vi "Dialog.vi"(8 "error in (no error)":errorcluster, 10 "latest tag":string, 11 "SelfUpdate in":refnum<class "SelfUpdate.lvclass">) -> (0 "error out":errorcluster, 2 "T button?":bool, 3 "SelfUpdate out":refnum<class "SelfUpdate.lvclass">)   [LabVIEW 2013, in "SelfUpdate.lvclass"]
uses:
  SelfUpdate.lvclass
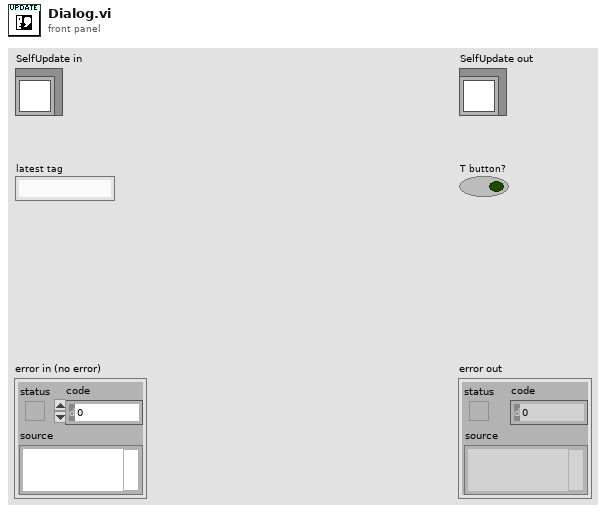
[diagram p1: front panel]
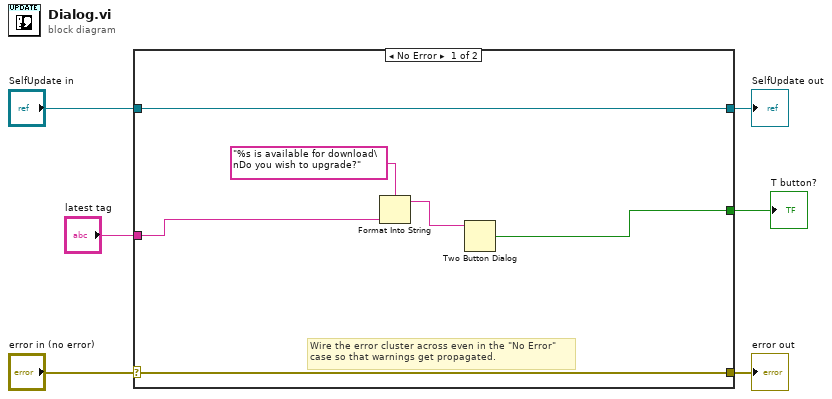
[diagram p0: block diagram]
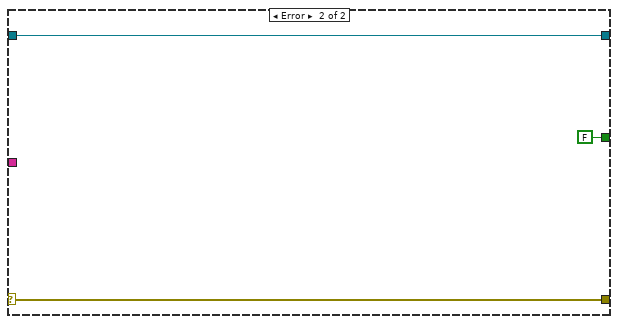
[diagram p2: hidden frame]
diagram:
  n1 = case shown="No Error" "error in (no error)" {
    selector: "error in (no error)" -> [w11 w15]
    tunnel: [w11 w15] -> w5
    tunnel: [w12 w14] -> w3
    tunnel: "SelfUpdate in" -> [w12 w14]
    tunnel: "latest tag" -> [w9 _]
    tunnel: [w7 FALSE ("T button?")] -> w1
    frame No Error {
      # "Wire the error cluster across even in the \"No Error\"\ncase so that warnings get propagated."
      n2 = Format Into String(format string="%s is available for download\nDo you wish to upgrade?" ("message"), w9) -> (resulting string=w8:string)  [unwired: 2 in, 1 out]
      n3 = Two Button Dialog(message=w8) -> (T button?=w7:bool)  [unwired: 2 in]
    }
    frame Error {
    }
  }
  "error out" <- w5
  "SelfUpdate out" <- w3
  "T button?" <- w1
